vi "Visa Write V2.vi"() -> ()   [LabVIEW 2022 SP3]
uses:
  <instrlib>/Keithley 2182/Keithley 2182.lvlib
  Keithley 24XX Sweep and Acquire Measurements Folder/Keithley 24XX.lvlib
panel:
  out "Buffer":dbl[](array[numeric])
  out "Resistance of DUT":dbl[](graph)
  out "Resistance (m-Ohms)":dbl[](array[numeric]) format="%.10f"
  in  "Sample Count To Display":i32=10
  out "Voltage Drop Across DUT":dbl[](graph)
  out "Delta Readings (uV)":ext[](array[numeric]) format="%.12f"
  in  "2182A":T1={"Baud Rate"=9600, "Parity"=0, "Data Bits"=8, "Stop Bits"=10, "Flow Control"=0, "VISA resource name"="SourceMeter2400"} {"Flow Control" items=["None", "XON/XOFF", "RTS/CTS", "XON/XOFF & RTS/CTS", "DTR/DSR", "XON/XOFF & DTR/DSR"]; "Stop Bits" items=["1.0"=10, "1.5"=15, "2.0"=20]; "Data Bits" items=["7"=7, "8"=8]; "Parity" items=["None", "Odd", "Even", "Mark", "Space"]; "Baud Rate" items=["300"=300, "600"=600, "1200"=1200, "2400"=2400, "4800"=4800, "9600"=9600, "19200"=19200]}
  in  "2400":T1={"Baud Rate"=9600, "Parity"=0, "Data Bits"=8, "Stop Bits"=10, "Flow Control"=0, "VISA resource name"="SourceMeter2400"} {"Flow Control" items=["None", "XON/XOFF", "RTS/CTS", "XON/XOFF & RTS/CTS", "DTR/DSR", "XON/XOFF & DTR/DSR"]; "Stop Bits" items=["1.0"=10, "1.5"=15, "2.0"=20]; "Data Bits" items=["7"=7, "8"=8]; "Parity" items=["None", "Odd", "Even", "Mark", "Space"]; "Baud Rate" items=["300"=300, "600"=600, "1200"=1200, "2400"=2400, "4800"=4800, "9600"=9600, "19200"=19200]}
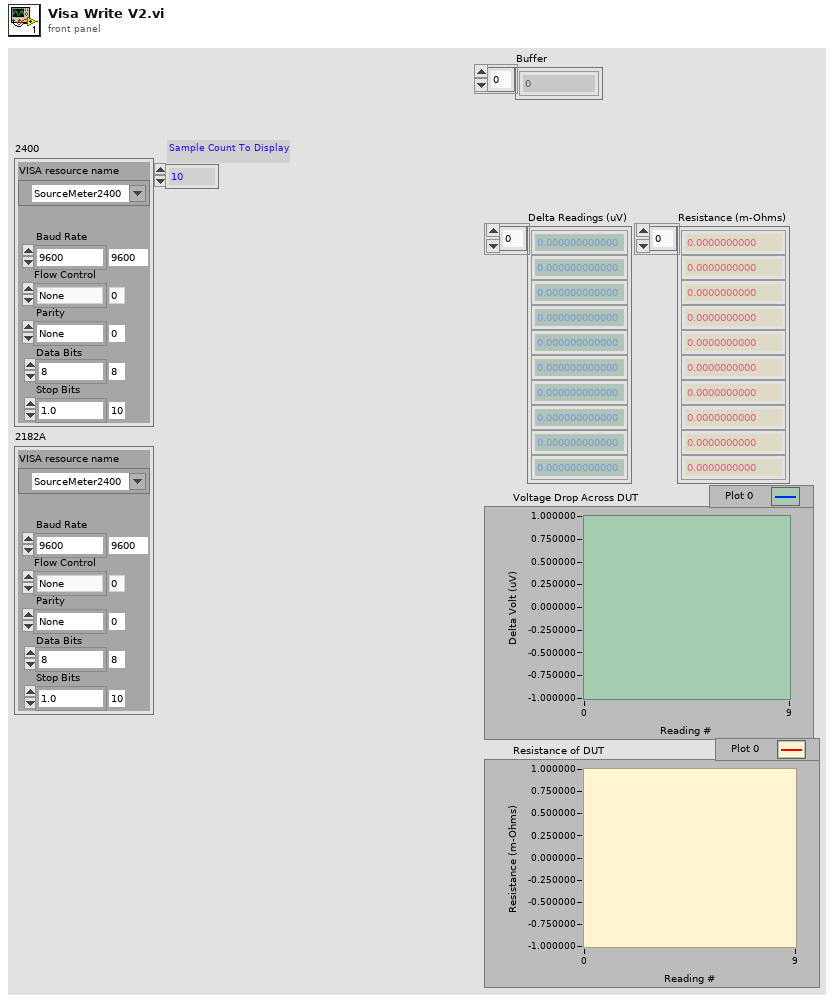
[diagram p1: front panel]
types:
  T1 = cluster{"Baud Rate":u32, "Parity":u16, "Data Bits":u16, "Stop Bits":u16, "Flow Control":u16, "VISA resource name":refnum<visa-resource-name>}
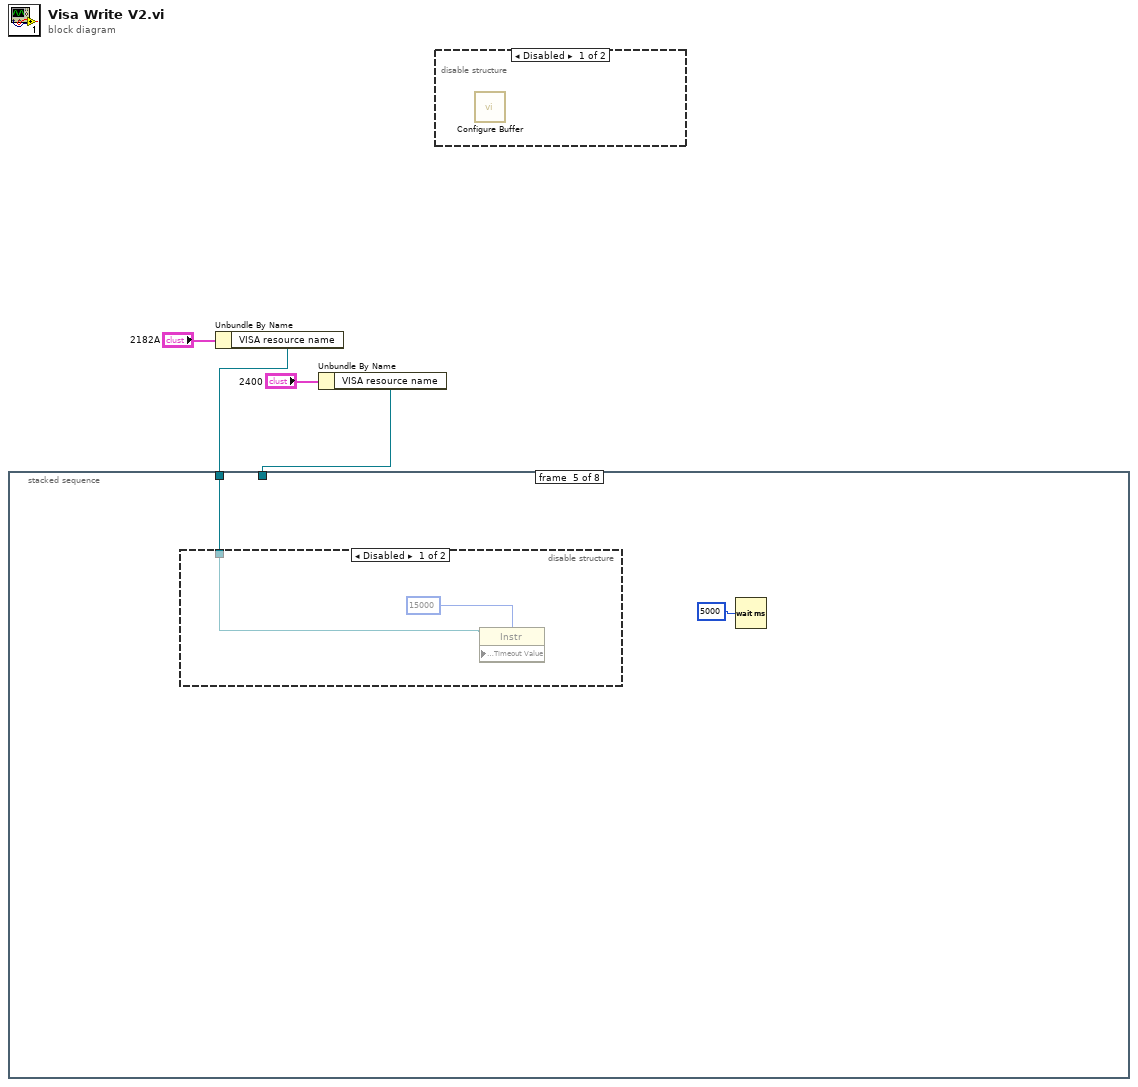
[diagram p0: block diagram]
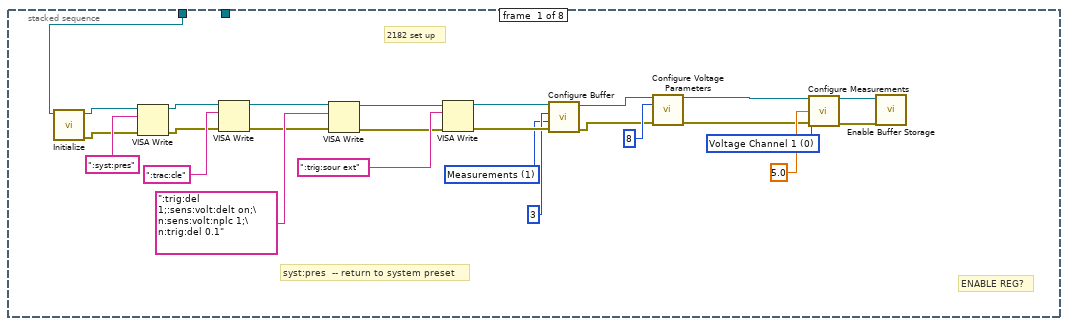
[diagram p3: hidden frame]
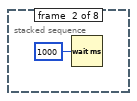
[diagram p4: hidden frame]
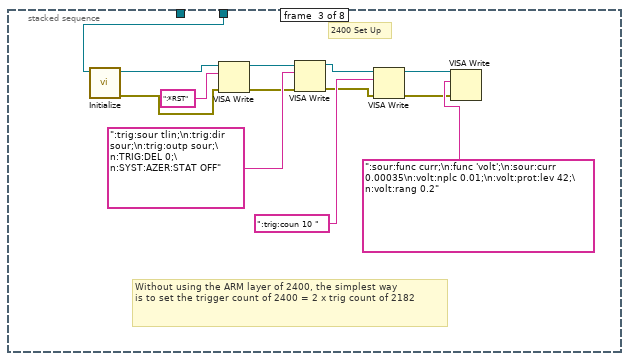
[diagram p5: hidden frame]
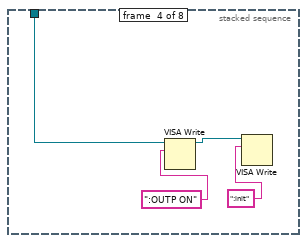
[diagram p6: hidden frame]
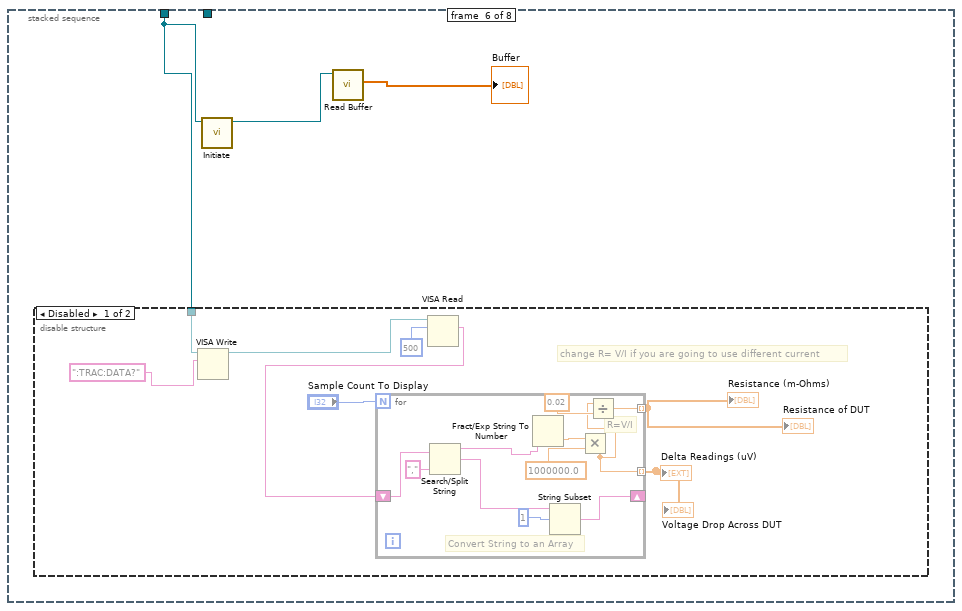
[diagram p8: hidden frame]
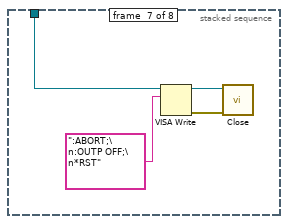
[diagram p10: hidden frame]
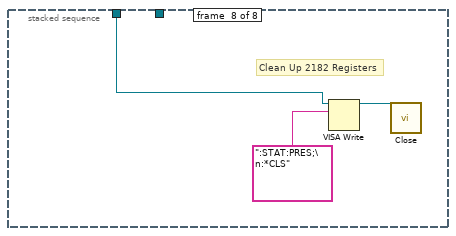
[diagram p11: hidden frame]
diagram:
  n1 = Unbundle By Name("2182A") -> ("VISA resource name"=w1:refnum<visa-resource-name>)
  n2 = Unbundle By Name("2400") -> ("VISA resource name"=w2:refnum<visa-resource-name>)
  n3 = stacked-sequence {
    tunnel: w1 -> [w23 _ _ _ w50 w54 _ w80]
    tunnel: w2 -> [_ _ w37 w48 _ _ w78 _]
    frame #0 {
      w5 = 1 items=["None", "Measurements", "Math Calculation"] ("Buffer Source (0: None)")
      w20 = 0 items=["Voltage Channel 1", "Voltage Channel 2", "Temperature Channel 1", "Temperature Channel 2"] ("Measurement (0: Voltage Channel 1)")
      # "ENABLE REG?"
      # "syst:pres  -- return to system preset"
      # "2182 set up"
      n4 = call <instrlib>:"Initialize.vi"("VISA resource name"=w23) -> ("error out"=w12:errorcluster, "VISA resource name out"=w22:refnum<visa-resource-name>)  [unwired: 9 in]
      n5 = VISA Write(VISA resource name=w22, write buffer=":syst:pres", error in (no error)=w12) -> (VISA resource name out=w24:refnum<visa-resource-name>, error out=w11:errorcluster)  [unwired: 1 out]
      n6 = VISA Write(VISA resource name=w24, write buffer=":trac:cle", error in (no error)=w11) -> (VISA resource name out=w26:refnum<visa-resource-name>, error out=w10:errorcluster)  [unwired: 1 out]
      n7 = VISA Write(VISA resource name=w26, write buffer=":trig:del 1;:sens:volt:delt on;\n:sens:volt:nplc 1;\n:trig:del 0.1", error in (no error)=w10) -> (VISA resource name out=w25:refnum<visa-resource-name>, error out=w9:errorcluster)  [unwired: 1 out]
      n8 = VISA Write(VISA resource name=w25, write buffer=":trig:sour ext", error in (no error)=w9) -> (VISA resource name out=w16:refnum<visa-resource-name>, error out=w14:errorcluster)  [unwired: 1 out]
      n9 = call <instrlib>:"Configure Buffer.vi"("error in (no error)"=w14, "Buffer Source (0: None)"=w5, "Buffer Size (2)"=3, "VISA resource name"=w16) -> ("error out"=w13:errorcluster, "VISA resource name out"=w15:refnum<visa-resource-name>)  [unwired: 6 in]
      n10 = call <instrlib>:"Configure Voltage Parameters.vi"("VISA resource name"=w15, "Voltage Resolution (8)"=8, "error in (no error)"=w13) -> ("VISA resource name out"=w21:refnum<visa-resource-name>, "error out"=w8:errorcluster)  [unwired: 11 in]
      n11 = call <instrlib>:"Configure Measurements.vi"("VISA resource name"=w21, "Measurement (0: Voltage Channel 1)"=w20, "Integration Rate (5)"=5.0, "error in (no error)"=w8) -> ("VISA resource name out"=w17:refnum<visa-resource-name>, "error out"=w7:errorcluster)  [unwired: 10 in]
      n12 = call <instrlib>:"Enable Buffer Storage.vi"("error in (no error)"=w7, "VISA resource name"=w17) -> ()  [unwired: 8 in, 2 out]
    }
    frame #1 {
      n13 = Wait (ms)(milliseconds to wait=u32 1000) -> ()  [unwired: 1 out]
    }
    frame #2 {
      # "Without using the ARM layer of 2400, the simplest way\nis to set the trigger count of 2400 = 2 x trig count of 2182"
      # "2400 Set Up"
      n14 = call <instrlib>:"Initialize.vi"("VISA resource name"=w37) -> ("error out"=w35:errorcluster, "VISA resource name out"=w36:refnum<visa-resource-name>)  [unwired: 9 in]
      n15 = VISA Write(VISA resource name=w36, write buffer=":*RST", error in (no error)=w35) -> (VISA resource name out=w44:refnum<visa-resource-name>, error out=w34:errorcluster)  [unwired: 1 out]
      n16 = VISA Write(VISA resource name=w44, write buffer=":trig:sour tlin;\n:trig:dir sour;\n:trig:outp sour;\n:TRIG:DEL 0;\n:SYST:AZER:STAT OFF", error in (no error)=w34) -> (VISA resource name out=w43:refnum<visa-resource-name>, error out=w33:errorcluster)  [unwired: 1 out]
      n17 = VISA Write(VISA resource name=w43, write buffer=":trig:coun 10 ", error in (no error)=w33) -> (VISA resource name out=w42:refnum<visa-resource-name>, error out=w32:errorcluster)  [unwired: 1 out]
      n18 = VISA Write(VISA resource name=w42, write buffer=":sour:func curr;\n:func 'volt';\n:sour:curr 0.00035\n:volt:nplc 0.01;\n:volt:prot:lev 42;\n:volt:rang 0.2", error in (no error)=w32) -> ()  [unwired: 3 out]
    }
    frame #3 {
      n19 = VISA Write(VISA resource name=w48, write buffer=":OUTP ON") -> (VISA resource name out=w47:refnum<visa-resource-name>)  [unwired: 1 in, 2 out]
      n20 = VISA Write(VISA resource name=w47, write buffer=":init") -> ()  [unwired: 1 in, 3 out]
    }
    frame #4 {
      n21 = disable-structure shown="Disabled" {
        disable-tunnel: w50 -> [w51 _]
        frame Disabled {
          n22 = property class="Instr"(reference=w51, "General Settings:Timeout Value"=u32 15000) -> ()  [unwired: 1 in, 2 out]
        }
        frame Enabled {
        }
      }
      n23 = Wait (ms)(milliseconds to wait=u32 5000) -> ()  [unwired: 1 out]
    }
    frame #5 {
      n24 = disable-structure shown="Disabled" {
        disable-tunnel: w54 -> [w62 _]
        frame Disabled {
          # "change R= V/I if you are going to use different current"
          n25 = VISA Write(VISA resource name=w62, write buffer=":TRAC:DATA?") -> (VISA resource name out=w56:refnum<visa-resource-name>)  [unwired: 1 in, 2 out]
          n26 = VISA Read(VISA resource name=w56, byte count=500) -> (read buffer=w57:string)  [unwired: 1 in, 3 out]
          n27 = for {
            N: "Sample Count To Display" -> [_]
            tunnel: [w65] -> w60 mode=indexing
            shift-right: [w70] -> _
            shift-left: w57 -> [w71]
            tunnel: [w67] -> w59 mode=indexing
            # "R=V/I"
            # "Convert String to an Array"
            n28 = Search/Split String(string=w71, search string/char (-)=",") -> (substring before match=w73:string, match + rest of string=w72:string)  [unwired: 1 in, 1 out]
            n29 = Fract/Exp String To Number(string=w73) -> (number=w64:dbl)  [unwired: 3 in, 1 out]
            n30 = String Subset(string=w72, offset (0)=1) -> (substring=w70:string)  [unwired: 1 in]
            n31 = Multiply(x=w64, y=1000000.0) -> (x*y=w65:dbl)
            n32 = Divide(x=w65, y=0.02 ("x")) -> (x/y=w67:dbl)
          }
          "Delta Readings (uV)" <- w60
          "Voltage Drop Across DUT" <- w60
          "Resistance (m-Ohms)" <- w59
          "Resistance of DUT" <- w59
        }
        frame Enabled {
        }
      }
      n33 = call <instrlib>:"Initiate.vi"("VISA resource name"=w54) -> ("VISA resource name out"=w53:refnum<visa-resource-name>)  [unwired: 9 in, 1 out]
      n34 = call <instrlib>:"Read Buffer.vi"("VISA resource name"=w53) -> ("Buffer"=→"Buffer":dbl[])  [unwired: 7 in, 3 out]
    }
    frame #6 {
      n35 = VISA Write(VISA resource name=w78, write buffer=":ABORT;\n:OUTP OFF;\n*RST" ("data")) -> (VISA resource name out=w76:refnum<visa-resource-name>, error out=w75:errorcluster)  [unwired: 1 in, 1 out]
      n36 = call <instrlib>:"Close.vi"("error in (no error)"=w75, "VISA resource name"=w76) -> ()  [unwired: 9 in, 1 out]
    }
    frame #7 {
      # "Clean Up 2182 Registers"
      n37 = VISA Write(VISA resource name=w80, write buffer=":STAT:PRES;\n:*CLS" ("data")) -> (VISA resource name out=w79:refnum<visa-resource-name>)  [unwired: 1 in, 2 out]
      n38 = call <instrlib>:"Close.vi"("VISA resource name"=w79) -> ()  [unwired: 10 in, 1 out]
    }
  }
  n39 = disable-structure shown="Disabled" {
    frame Disabled {
      n40 = call <instrlib>:"Configure Buffer.vi"() -> ()  [unwired: 10 in, 2 out]
    }
    frame Enabled {
    }
  }
